vi "Enqueue.vi"(7 "Priority(?) (f)":bool, 8 "ErrorArray":errorcluster[](array[cluster]), 9 "Data":variant, 10 "Message":string) -> (0 "ErrorArray":errorcluster[](array[cluster]))   [LabVIEW 2014, in "TestBase.lvclass"]
uses:
  TestBase.lvclass
  clQueMsgType.ctl
  <userlib>/NIST/NISTErrorLib/NISTErrorLib.lvlib
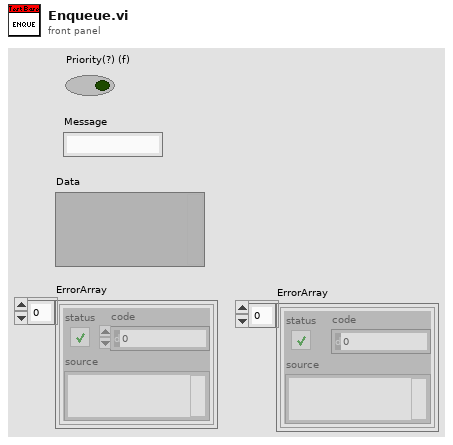
[diagram p1: front panel]
types:
  T1 = typedef "TestBase.lvclass/clQueMsgType.ctl" = cluster{"Message":string, "Data":variant}
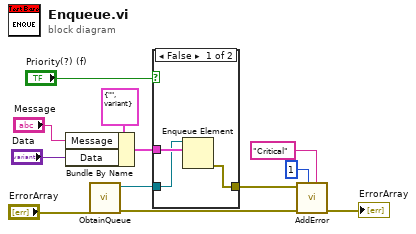
[diagram p0: block diagram]
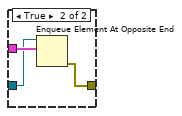
[diagram p2: hidden frame]
diagram:
  n1 = Bundle By Name(cluster=T1 {"Message"="", "Data"=variant} ("clQueMsgType"), "Message"="Message", "Data"="Data") -> (w7:T1)
  n2 = call "ObtainQueue.vi"("ErrorArray"="ErrorArray") -> ("ErrorArray."=w4:errorcluster[], "TstQue"=w3:refnum<queue>)  [unwired: 9 in]
  n3 = case shown="False" "Priority(?) (f)" {
    tunnel: w7 -> [w14 w18]
    tunnel: w3 -> [w13 w17]
    tunnel: [w15 w16] -> w2
    frame False {
      n4 = Enqueue Element(queue=w13, element=w14) -> (error out=w15:errorcluster)  [unwired: 2 in, 2 out]
    }
    frame True {
      n5 = Enqueue Element At Opposite End(queue=w17, element=w18) -> (error out=w16:errorcluster)  [unwired: 2 in, 2 out]
    }
  }
  n6 = call <userlib>:"AddError.vi"("Severity"="Critical", "Priority"=u8 1, "ErrorArray"=w4, "error in (no error)"=w2) -> ("ErrorArray"=→"ErrorArray":errorcluster[])  [unwired: 6 in, 1 out]
